vi "历史数据记录.vi"(0 "成员信息":string, 1 "?":bool, 2 "心率":dbl, 3 "收缩压":dbl, 4 "舒张压":dbl) -> ()   [LabVIEW 2016]
uses:
  <vilib>/Utility/file.llb/Read Delimited Spreadsheet (I64).vi
  <vilib>/Utility/file.llb/Write Delimited Spreadsheet (I64).vi
  <vilib>/Utility/file.llb/Write Delimited Spreadsheet (DBL).vi
panel:
  in  "1D data":dbl[](array[numeric]) caption="一维数据"
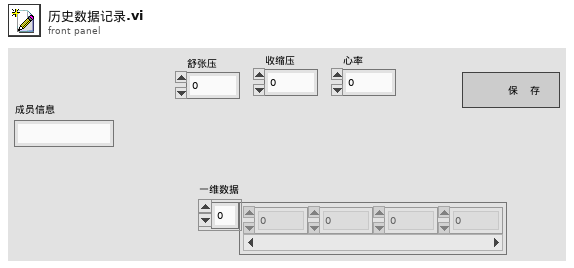
[diagram p1: front panel]
types:
  T1 = typedef "LVDateTimeRec.ctl" = cluster{"秒数的小数部分":dbl, "秒":i32, "分":i32, "时":i32, "日":i32, "月":i32, "年":i32, "天数（周）":i32, "天数（年）":i32, "DST":i32}
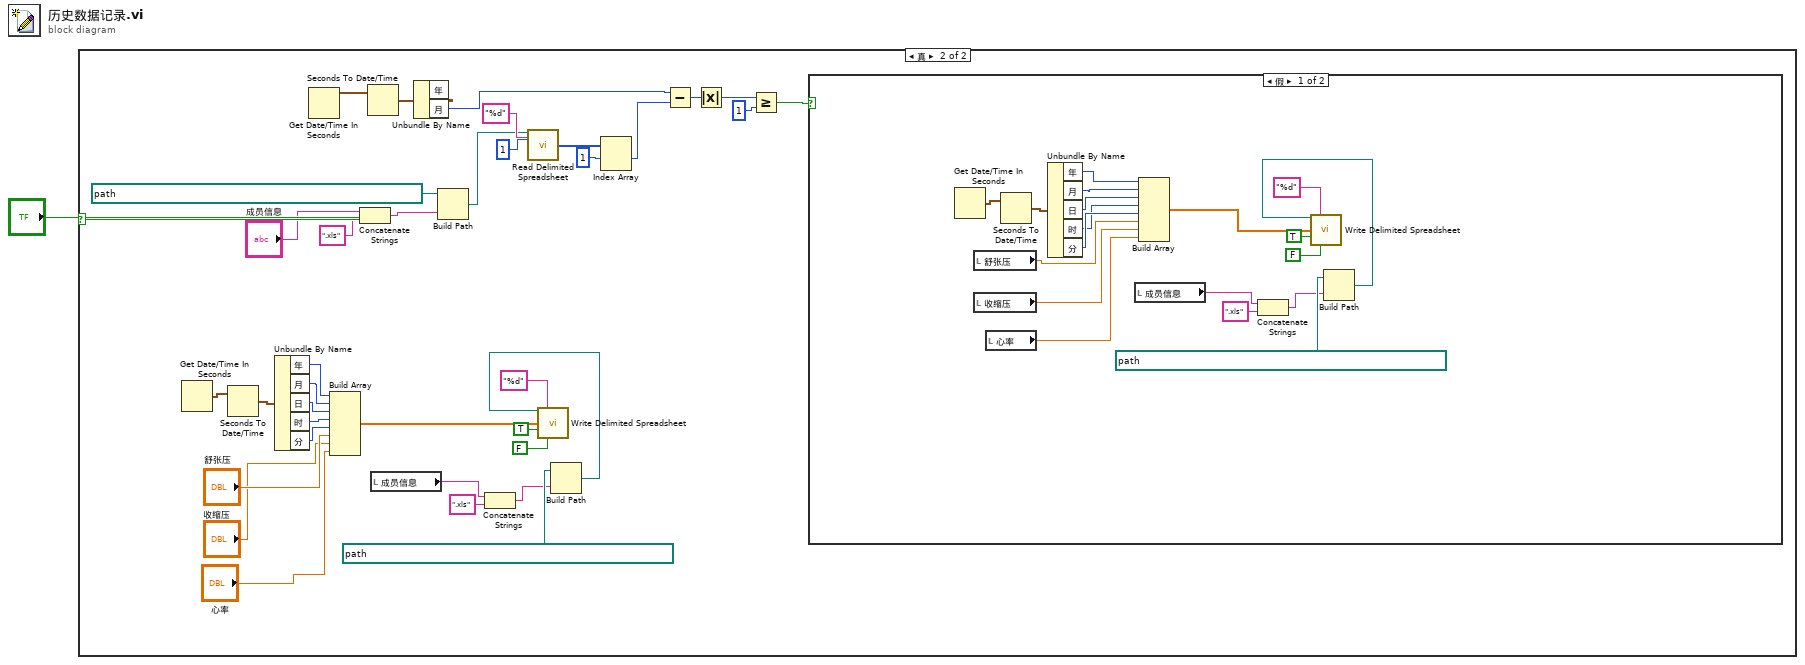
[diagram p0: block diagram]
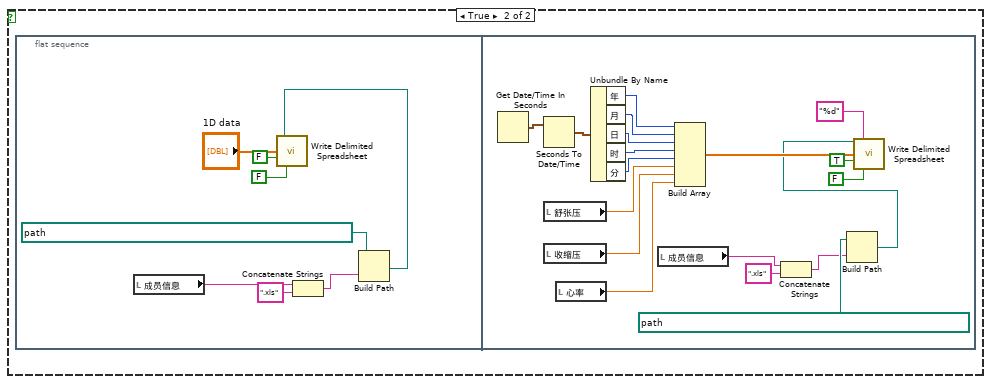
[diagram p3: hidden frame]
diagram:
  n1 = case shown="真" "?" {
    frame False {
    }
    frame True {
      n2 = Get Date/Time In Seconds() -> (seconds since 1Jan1904=w20:timestamp)
      n3 = Seconds To Date/Time(time stamp (now)=w20) -> (date time rec=w19:T1)  [unwired: 1 in]
      n4 = Unbundle By Name(w19) -> ("年"=w15:i32, "月"=w10:i32, "日"=w16:i32, "时"=w17:i32, "分"=w18:i32)
      n5 = Get Date/Time In Seconds() -> (seconds since 1Jan1904=w37:timestamp)
      n6 = Build Array(w15, w10, w16, w17, w18, "舒张压", "收缩压", "心率") -> (w14:dbl[])
      n7 = Concatenate Strings("成员信息", ".xls" ("字符串")) -> (w24:string)
      n8 = Seconds To Date/Time(time stamp (now)=w37) -> (date time rec=w36:T1)  [unwired: 1 in]
      n9 = local read "成员信息"() -> (w2:string)
      n10 = Unbundle By Name(w36) -> ("月"=w21:i32)  [unwired: 1 out]
      n11 = Build Path(base path=path "C:/Users/Administrator/Desktop/课程设计/本月数据记录" ("基路径"), name or relative path=w24) -> (appended path=w23:path)
      n12 = Concatenate Strings(w2, ".xls" ("字符串")) -> (w7:string)
      n13 = call-poly <vilib>:"Read Delimited Spreadsheet.vi"("file path (dialog if empty)"=w23, "format (%d)"="%d", "number of rows (all:-1)"=1) -> ("first row"=w34:i64[])  [unwired: 7 in, 5 out]
      n14 = Build Path(base path=path "C:/Users/Administrator/Desktop/课程设计/历史数据记录" ("基路径"), name or relative path=w7) -> (appended path=w6:path)
      n15 = call-poly <vilib>:"Write Delimited Spreadsheet.vi"("file path (dialog if empty)"=w6, "format (%d)"="%d" ("format (%.3f)"), "1D data"=w14, "append to file? (new file:F)"=TRUE, "transpose? (no:F)"=FALSE) -> ()  [unwired: 9 in, 2 out]
      n16 = Index Array(array=w34, index #1=1 ("索引")) -> (element #1=w32:i64)  [unwired: 1 in, 1 out]
      n17 = Subtract(x=w21, y=w32) -> (x-y=w29:i64)
      n18 = Absolute Value(x=w29) -> (abs(x)=w28:i64)
      n19 = Greater Or Equal?(x=w28, y=i64 1) -> (x >= y?=w30:bool)
      n20 = case shown="假" w30 {
        frame False {
          n21 = Get Date/Time In Seconds() -> (seconds since 1Jan1904=w56:timestamp)
          n22 = local read "舒张压"() -> (w40:dbl)
          n23 = local read "收缩压"() -> (w39:dbl)
          n24 = local read "心率"() -> (w38:dbl)
          n25 = Seconds To Date/Time(time stamp (now)=w56) -> (date time rec=w55:T1)  [unwired: 1 in]
          n26 = Unbundle By Name(w55) -> ("年"=w51:i32, "月"=w46:i32, "日"=w52:i32, "时"=w53:i32, "分"=w54:i32)
          n27 = local read "成员信息"() -> (w41:string)
          n28 = Build Array(w51, w46, w52, w53, w54, w40, w39, w38) -> (w50:dbl[])
          n29 = Concatenate Strings(w41, ".xls" ("字符串")) -> (w43:string)
          n30 = Build Path(base path=path "C:/Users/Administrator/Desktop/课程设计/本月数据记录" ("基路径"), name or relative path=w43) -> (appended path=w42:path)
          n31 = call-poly <vilib>:"Write Delimited Spreadsheet.vi"("file path (dialog if empty)"=w42, "format (%d)"="%d" ("format (%.3f)"), "1D data"=w50, "append to file? (new file:F)"=TRUE, "transpose? (no:F)"=FALSE) -> ()  [unwired: 9 in, 2 out]
        }
        frame True {
          n32 = flat-sequence {
            frame #0 {
              n33 = local read "成员信息"() -> (w59:string)
              n34 = Concatenate Strings(w59, ".xls" ("字符串")) -> (w61:string)
              n35 = Build Path(base path=path "C:/Users/Administrator/Desktop/课程设计/本月数据记录" ("基路径"), name or relative path=w61) -> (appended path=w60:path)
              n36 = call-poly <vilib>:"Write Delimited Spreadsheet.vi"("file path (dialog if empty)"=w60, "1D data"="1D data", "append to file? (new file:F)"=FALSE, "transpose? (no:F)"=FALSE) -> ()  [unwired: 10 in, 2 out]
            }
            frame #1 {
              n37 = Get Date/Time In Seconds() -> (seconds since 1Jan1904=w83:timestamp)
              n38 = Seconds To Date/Time(time stamp (now)=w83) -> (date time rec=w82:T1)  [unwired: 1 in]
              n39 = local read "舒张压"() -> (w67:dbl)
              n40 = local read "收缩压"() -> (w66:dbl)
              n41 = local read "心率"() -> (w65:dbl)
              n42 = Unbundle By Name(w82) -> ("年"=w78:i32, "月"=w73:i32, "日"=w79:i32, "时"=w80:i32, "分"=w81:i32)
              n43 = local read "成员信息"() -> (w68:string)
              n44 = Build Array(w78, w73, w79, w80, w81, w67, w66, w65) -> (w77:dbl[])
              n45 = Concatenate Strings(w68, ".xls" ("字符串")) -> (w70:string)
              n46 = Build Path(base path=path "C:/Users/Administrator/Desktop/课程设计/本月数据记录" ("基路径"), name or relative path=w70) -> (appended path=w69:path)
              n47 = call-poly <vilib>:"Write Delimited Spreadsheet.vi"("file path (dialog if empty)"=w69, "format (%d)"="%d" ("format (%.3f)"), "1D data"=w77, "append to file? (new file:F)"=TRUE, "transpose? (no:F)"=FALSE) -> ()  [unwired: 9 in, 2 out]
            }
          }
        }
      }
    }
  }
